vi "Callback Change UA Data Type.vi"(6 "Variant":variant, 8 "error in (no error)":errorcluster, 9 "old values":string[][](array[string]), 10 "object ref in":T2, 11 "Cluster":T3) -> (0 "error out":errorcluster)   [LabVIEW 2014, in "OPC UA Client editor node.lvclass"]
uses:
  OPC UA Client editor node.lvclass
  <vilib>/NI/DCAF/Tag Editor Core/Table API/Table Manager/Cell Change.ctl
  <vilib>/NI/DCAF/Tag Editor Core/Table API/Table Manager/object ref.ctl
  <vilib>/NI/DCAF/Tag Editor Core/Configuration Editor/Classes/Engine Parent/Engine Parent Editor Node.lvclass
  <vilib>/NI/DCAF/Tag Editor Core/Configuration Editor/Classes/Module editor node/module editor node.lvclass
  OPC UA DataType Enum.ctl
  module/configuration/OPC UA Client configuration.lvclass
  module/configuration/OPC UA Client configuration.lvclass/OPC UA Client configuration.ctl
  <vilib>/NI/Tag Bus/tag/tag descriptor.lvclass/tag descriptor.ctl
  <vilib>/NI/Tag Bus Module Framework/channel/TBM channel.lvclass
  <vilib>/NI/DCAF/Tag Editor Core/Table API/Table Manager.lvlib
  <vilib>/NI/Tag Bus/tag/tag descriptor.lvclass
  <vilib>/NI/DCAF/Tag Editor Core/Table API/Table Manager/Table Manager.lvclass
panel:
  in  "data type":T1
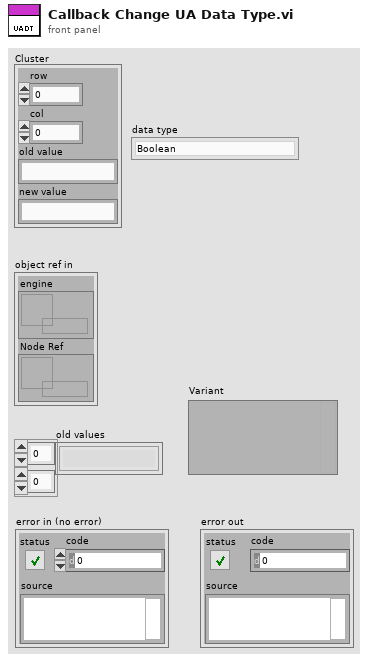
[diagram p1: front panel]
types:
  T1 = typedef "OPC UA Client editor node.lvclass/OPC UA DataType Enum.ctl" = enum16{"Boolean", "SByte", "Byte", "Int16", "UInt16", "Int32", "UInt32", "Int64", "UInt64", "Float", "Double", "String", "DateTime", "ByteString", "Array of Boolean", "Array of SByte", "Array of Byte", "Array of Int16", "Array of UInt16", "Array of Int32", "Array of UInt32", "Array of Int64", "Array of UInt64", "Array of Float", "Array of Double", "Array of String", "Array of DateTime"}
  T2 = typedef "Table Manager.lvlib/Table Manager.lvclass/object ref.ctl" = cluster{"engine":refnum<data-value>, "Node Ref":refnum<data-value>}
  T3 = typedef "Table Manager.lvlib/Cell Change.ctl" = cluster{"row":i32, "col":i32, "old value":string, "new value":string}
  T4 = typedef "OPC UA Client configuration.lvclass/Line.ctl" = cluster{"channel":refnum<class "TBM channel.lvclass">, "Node Path":string, "OPC UA Data Type":T5}
  T5 = typedef "OPC UA Client configuration.lvclass/OPC UA Data Type.ctl" = u16
  T6 = typedef "tag bus.lvlib/tag descriptor.lvclass/Data Type.ctl" = enum16{"Double", "Single", "I64", "I32", "I16", "I8", "U64", "U32", "U16", "U8", "Boolean", "String", "Array of Double", "Array of Single", "Array of I64", "Array of I32", "Array of I16", "Array of I8", "Array of U64", "Array of U32", "Array of U16", "Array of U8", "Array of Boolean", "Array of String"}
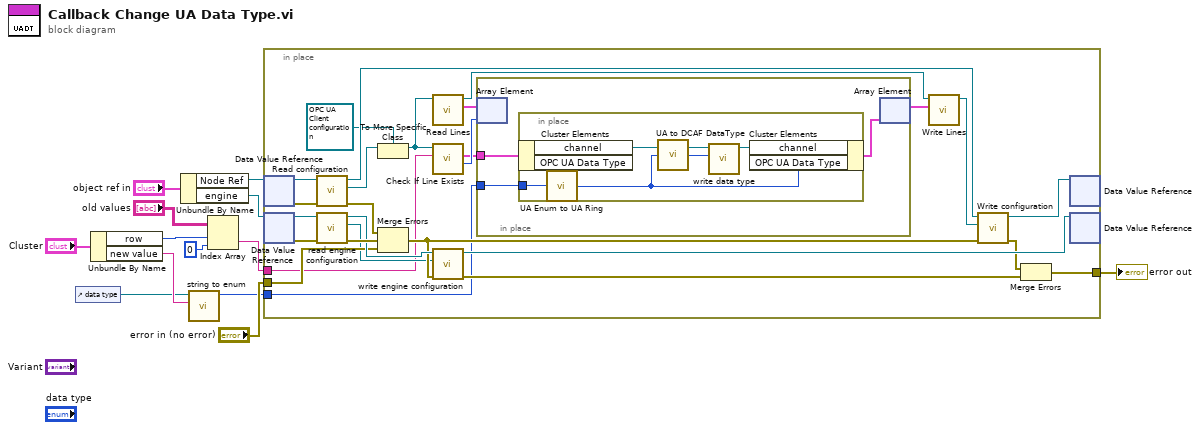
[diagram p0: block diagram]
diagram:
  n1 = control-ref of="data type"() -> (w1:refnum<vi>)
  n2 = Unbundle By Name("Cluster") -> ("row"=w5:i32, "new value"=w3:string)
  n3 = Unbundle By Name("object ref in") -> ("Node Ref"=w10:refnum<data-value>, "engine"=w9:refnum<data-value>)
  n4 = call <vilib>:"string to enum.vi"("String"=w3, "Enum"=w1) -> ("Value"=w2:i32)  [unwired: 8 in, 1 out]
  n5 = Index Array(array="old values", index (row)=w5, index (col)=0 ("disabled index (col)")) -> (element=w4:string)
  n6 = in-place {
    in-place-border: [w32] -> w13
    in-place-border: "error in (no error)" -> [w25]
    in-place-border: w4 -> [w16]
    in-place-border: w2 -> [w14]
    n7 = in-place-dvr #1(w10) -> (w29:refnum<class "module editor node.lvclass">, w31:errorcluster)
    n8 = in-place-dvr #2(w9) -> (w39:refnum<class "Engine Parent Editor Node.lvclass">, w40:errorcluster)
    n9 = call-dynamic "Read configuration.vi"("error in"=w31, "NISE_CEF_serializable node in"=w29) -> ("error out"=w30:errorcluster, "configuration"=w27:refnum<class "NISE_CEF_serializable configuration.lvclass">, "NISE_CEF_serializable node out"=w28:refnum<class "module editor node.lvclass">)  [unwired: 7 in]
    n10 = call <vilib>:"read engine configuration.vi"("error in"=w40, "Engine Parent Editor Node in"=w39) -> ("error out"=w36:errorcluster, "engine configuration"=w24:refnum<class "engine configuration.lvclass">, "Engine Parent Editor Node out"=w35:refnum<class "Engine Parent Editor Node.lvclass">)  [unwired: 7 in]
    n11 = To More Specific Class(target class=refnum<class "OPC UA Client configuration.lvclass"> refnum ("tag bus configurable plugin module configuration"), reference=w27) -> (specific class reference=w20:refnum<class "OPC UA Client configuration.lvclass">)  [unwired: 1 in, 1 out]
    n12 = Merge Errors(w30, w36, w25) -> (w26:errorcluster)
    n13 = call "Read Lines.vi"("OPC UA configuration in"=w20) -> ("Lines"=w19:T4[], "OPC UA configuration out"=w21:refnum<class "OPC UA Client configuration.lvclass">)  [unwired: 8 in, 1 out]
    n14 = call-dynamic "Check If Line Exists.vi"("name to locate"=w16, "OPC UA configuration in"=w20) -> ("index"=w17:i32, "Line out"=w15:T4)  [unwired: 5 in, 3 out]
    n15 = call <vilib>:"write engine configuration.vi"("error in"=w26, "engine configuration"=w24, "Engine Parent Editor Node in"=w35) -> ("error out"=w34:errorcluster, "Engine Parent Editor Node out"=w38:refnum<class "Engine Parent Editor Node.lvclass">)  [unwired: 7 in]
    n16 = in-place {
      in-place-border: w15 -> [w43]
      in-place-border: w14 -> [w42]
      n17 = in-place-array #3(w19, w17) -> ()  [unwired: 1 out]
      n18 = in-place {
        in-place-border: w42 -> [w46]
        n19 = in-place-cluster #4(w43) -> ("channel"=w48:refnum<class "TBM channel.lvclass">)  [unwired: 1 out]
        n20 = call "UA Enum to UA Ring.vi"("OPC Data Type Enum"=w46) -> ("OPC UA Data Type Ring"=w44:T5)
        n21 = call "UA to DCAF DataType.vi"("OPC UA Data Type"=w44) -> ("DCAF Datatype"=w45:T6)
        n22 = call <vilib>:"write data type.vi"("data type"=w45, "system tag in"=w48) -> ("system tag out"=w47:refnum<class "TBM channel.lvclass">)  [unwired: 8 in, 1 out]
        n23 = in-place-cluster #4("channel"=w47, "OPC UA Data Type"=w44) -> (w41:T4)
      }
      n24 = in-place-array #3(w41) -> (w18:T4[])  [unwired: 1 out]
    }
    n25 = call "Write Lines.vi"("Lines"=w18, "OPC UA configuration in"=w21) -> ("OPC UA configuration out"=w22:refnum<class "OPC UA Client configuration.lvclass">)  [unwired: 8 in, 1 out]
    n26 = call-dynamic "Write configuration.vi"("error in"=w26, "configuration"=w22, "NISE_CEF_serializable node in"=w28) -> ("error out"=w33:errorcluster, "NISE_CEF_serializable node out"=w37:refnum<class "module editor node.lvclass">)  [unwired: 7 in]
    n27 = Merge Errors(w33, w34) -> (w32:errorcluster)
    n28 = in-place-dvr #1(w37) -> ()  [unwired: 2 out]
    n29 = in-place-dvr #2(w38) -> ()  [unwired: 2 out]
  }
  "error out" <- w13
